vi "TimeTransform.vi"(0 "Speed Y":dbl, 4 "Speed X":dbl, 6 "Speed Scale":dbl, 8 "Speed Rotate":dbl, 9 "Elapsed Time":u32, 10 "Y":u32[](array[numeric]), 11 "X":u32[](array[numeric])) -> (2 "Y out":u32[](array[numeric]), 3 "X out":u32[](array[numeric]))   [LabVIEW 2017, in "AODControl.lvlib"]
uses:
  AODControl.lvlib
  <vilib>/Analysis/coordinate.llb/2D Cartesian Coordinate Rotation (Array).vi
  DecodifyFrequency(Array).vi
  CodifyFrequency(Array).vi
  <vilib>/Analysis/NI_AALPro.lvlib
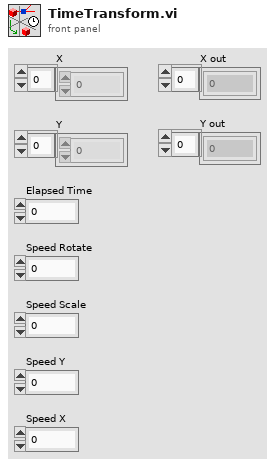
[diagram p1: front panel]
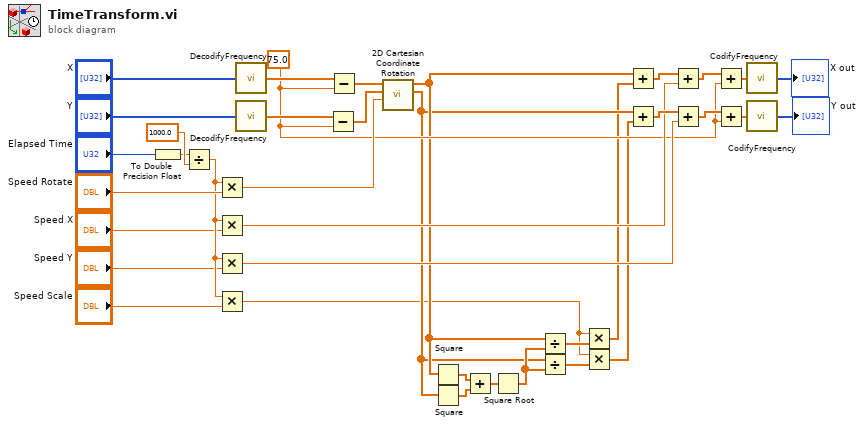
[diagram p0: block diagram]
diagram:
  w12 = 75.0
  n1 = To Double Precision Float(number="Elapsed Time") -> (double precision float=w28:dbl)
  n2 = Divide(x=w28, y=1000.0) -> (x/y=w24:dbl)
  n3 = Multiply(x=w24, y="Speed Rotate") -> (x*y=w35:dbl)
  n4 = Multiply(x=w24, y="Speed X") -> (x*y=w19:dbl)
  n5 = Multiply(x=w24, y="Speed Y") -> (x*y=w18:dbl)
  n6 = Multiply(x=w24, y="Speed Scale") -> (x*y=w1:dbl)
  n7 = call-poly "DecodifyFrequency.vi"("Array 2"="X") -> ("Array"=w31:dbl[])
  n8 = call-poly "DecodifyFrequency.vi"("Array 2"="Y") -> ("Array"=w32:dbl[])
  n9 = Subtract(x=w32, y=w12) -> (x-y=w34:dbl[])
  n10 = Subtract(x=w31, y=w12) -> (x-y=w33:dbl[])
  n11 = call-poly <vilib>:"2D Cartesian Coordinate Rotation.vi"("theta"=w35, "Y"=w34, "X"=w33) -> ("Y Out"=w6:dbl[], "X Out"=w7:dbl[])  [unwired: 6 in, 1 out]
  n12 = Square(x=w7) -> (x^2=w11:dbl[])
  n13 = Square(x=w6) -> (x^2=w10:dbl[])
  n14 = Add(x=w11, y=w10) -> (x+y=w9:dbl[])
  n15 = Square Root(x=w9) -> (sqrt(x)=w8:dbl[])
  n16 = Divide(x=w7, y=w8) -> (x/y=w5:dbl[])
  n17 = Divide(x=w6, y=w8) -> (x/y=w4:dbl[])
  n18 = Multiply(x=w1, y=w5) -> (x*y=w3:dbl[])
  n19 = Multiply(x=w1, y=w4) -> (x*y=w2:dbl[])
  n20 = Add(x=w7, y=w3) -> (x+y=w23:dbl[])
  n21 = Add(x=w6, y=w2) -> (x+y=w22:dbl[])
  n22 = Add(x=w23, y=w19) -> (x+y=w16:dbl[])
  n23 = Add(x=w22, y=w18) -> (x+y=w15:dbl[])
  n24 = Add(x=w16, y=w12) -> (x+y=w13:dbl[])
  n25 = Add(x=w15, y=w12) -> (x+y=w14:dbl[])
  n26 = call-poly "CodifyFrequency.vi"("Array"=w13) -> ("Array 2"=→"X out":u32[])
  n27 = call-poly "CodifyFrequency.vi"("Array"=w14) -> ("Array 2"=→"Y out":u32[])
